vi "Person_Create.vi"(0 "Name":string, 5 "ISpeakBehaviour":refnum<class "ISpeakBehaviour.lvclass">, 7 "ILearnBehaviour":refnum<class "ILearnBehaviour.lvclass">, 9 "PicturePath":path, 11 "Error In":errorcluster) -> (4 "reference out":refnum<class "Person.lvclass">, 15 "Error Out":errorcluster)   [LabVIEW 2024, in "Person.lvclass"]
uses:
  Person.lvclass
  ILearnBehaviour/ILearnBehaviour.lvclass
  ISpeakBehaviour/ISpeakBehaviour.lvclass
  Person.lvclass/Person.ctl
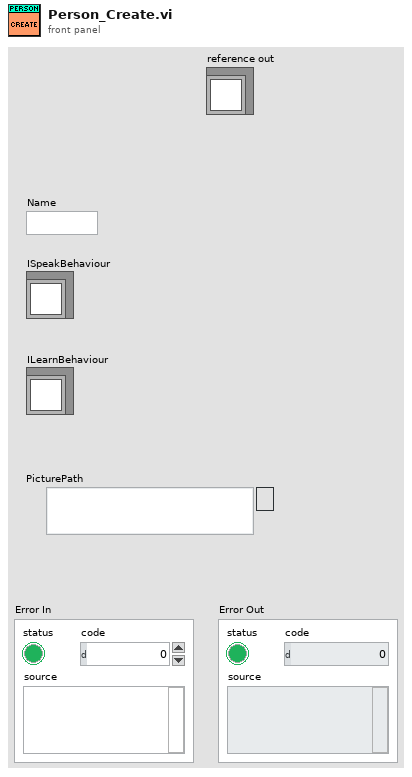
[diagram p1: front panel]
types:
  T1 = typedef "Person.lvclass/ObjectAttributes.ctl" = cluster{"SpeakBehaviour":refnum<class "ISpeakBehaviour.lvclass">, "LearnBehaviour":refnum<class "ILearnBehaviour.lvclass">, "Name":string, "PicturePath":path}
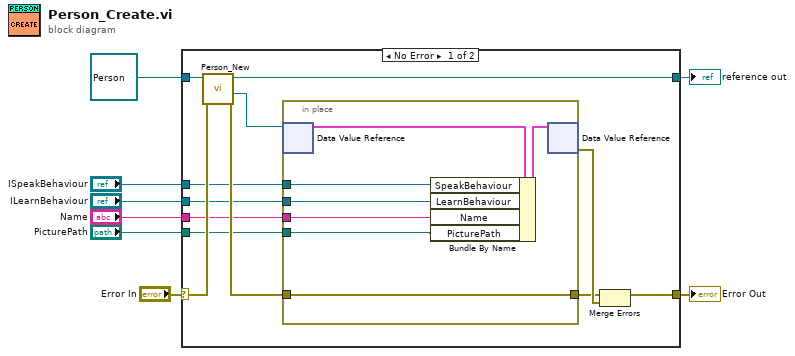
[diagram p0: block diagram]
diagram:
  n1 = case shown="No Error" "Error In" {
    selector: "Error In" -> [w19 w29]
    tunnel: [w13 w29] -> w7
    tunnel: refnum<class "Person.lvclass"> refnum ("reference in") -> [w20 w28]
    tunnel: [w18 w28] -> w5
    tunnel: "ILearnBehaviour" -> [w12 _]
    tunnel: "ISpeakBehaviour" -> [w11 _]
    tunnel: "Name" -> [w10 _]
    tunnel: "PicturePath" -> [w9 _]
    frame No Error {
      n2 = call "Person_New.vi"("Error In"=w19, "reference in"=w20) -> ("Error Out"=w15:errorcluster, "DVRRefOut"=w16:refnum<data-value>, "reference out"=w18:refnum<class "Person.lvclass">)  [unwired: 6 in, 1 out]
      n3 = in-place {
        in-place-border: w15 -> [w25]
        in-place-border: [w25] -> w14
        in-place-border: w12 -> [w24]
        in-place-border: w11 -> [w23]
        in-place-border: w10 -> [w22]
        in-place-border: w9 -> [w21]
        n4 = in-place-dvr #1(w16) -> (w26:T1)  [unwired: 1 out]
        n5 = Bundle By Name(cluster=w26, "SpeakBehaviour"=w23, "LearnBehaviour"=w24, "Name"=w22, "PicturePath"=w21) -> (w27:T1)
        n6 = in-place-dvr #1(w27) -> (w17:errorcluster)  [unwired: 1 out]
      }
      n7 = Merge Errors(w14, w17) -> (w13:errorcluster)
    }
    frame Error {
      # "VI-TechBaseTemplate_Simple_4x4x4"
    }
  }
  "Error Out" <- w7
  "reference out" <- w5
